vi "检查配置文件引用.vi"(8 "error in (no error)":errorcluster caption="错误输入（无错误）", 11 "启动器 输入":refnum<class "启动器.lvclass">) -> (0 "error out":errorcluster caption="错误输出", 2 "无效?":bool, 3 "启动器 输出":refnum<class "启动器.lvclass">)   [LabVIEW 2017, in "启动器.lvlib" / "启动器.lvclass"]
doc: "有效为 F, \n无效为 T."
uses:
  <vilib>/Utility/config.llb/NI_LVConfig.lvlib
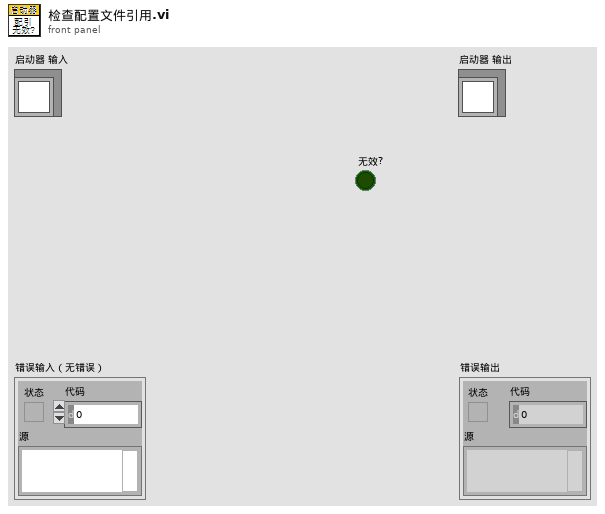
[diagram p1: front panel]
types:
  T1 = typedef "NI_LVConfig.lvlib/Config Data RefNum.ctl" = refnum<k1>
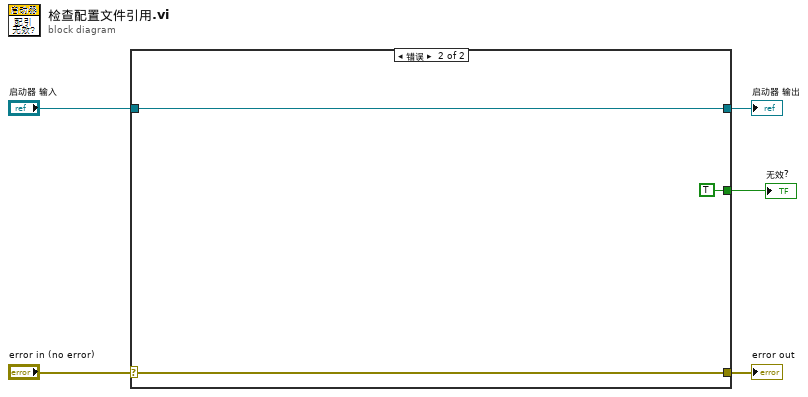
[diagram p0: block diagram]
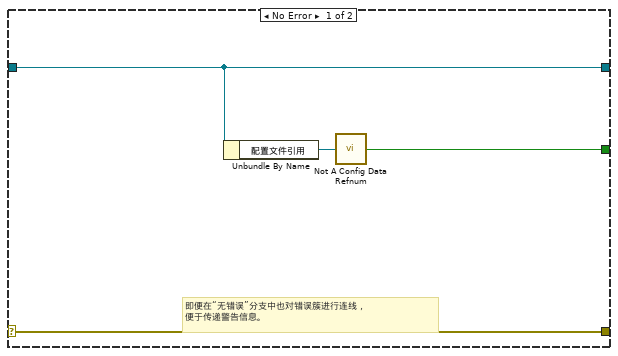
[diagram p2: hidden frame]
diagram:
  n1 = case shown="错误" "error in (no error)" {
    selector: "error in (no error)" -> [w9 w12]
    tunnel: [w9 w12] -> w4
    tunnel: [w8 w11] -> w2
    tunnel: "启动器 输入" -> [w8 w11]
    tunnel: [w6 TRUE ("not a config data refnum")] -> w1
    frame No Error {
      # "即便在“无错误”分支中也对错误簇进行连线，\n便于传递警告信息。"
      n2 = Unbundle By Name(w8) -> ("配置文件引用"=w7:T1)
      n3 = call <vilib>:"Not A Config Data Refnum.vi"("refnum"=w7) -> ("not a config data refnum"=w6:bool)
    }
    frame Error {
    }
  }
  "error out" <- w4
  "启动器 输出" <- w2
  "无效?" <- w1
